vi "Type Conv - Dryer Status to Txt.vi"(11 "Status":T1) -> (3 "Ring Text.Text":string)   [LabVIEW 2012]
uses:
  Dryer Status Ctrl.ctl
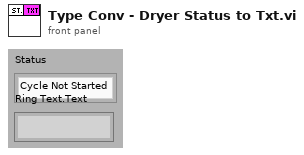
[diagram p1: front panel]
types:
  T1 = typedef "Dryer Status Ctrl.ctl" = enum16{"Cycle Not Started", "Cycle Running", "Paused", "Cycle Completed", "Eval Mode Entered", "Err", "Pause (No GEA2)"}
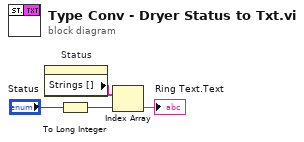
[diagram p0: block diagram]
diagram:
  n1 = property on="Status" class="Enum (strict)"() -> ("Strings []"=w4:string[])  [unwired: 2 in, 2 out]
  n2 = To Long Integer(number="Status") -> (32bit integer=w2:i32)
  n3 = Index Array(array=w4, index=w2) -> (element=→"Ring Text.Text":string)
